vi "Field Transform Joystick.vi"(7 "use field orientation":bool, 9 "Climber Angle":bool, 10 "robot field orientation (deg)":dbl, 11 "Joystick Values":dbl[](array[numeric])) -> (3 "Transformed Joystick Values":dbl[](array[numeric]))   [LabVIEW 2019]
uses:
  <vilib>/Analysis/coordinate.llb/2D Cartesian Coordinate Rotation (Scalar).vi
  <vilib>/addons/control/pid/pid.llb/PID (DBL).vi
  <vilib>/Rock Robotics/Network Tables/NT Write Boolean.vi
  <vilib>/Analysis/NI_AALPro.lvlib
  <vilib>/addons/control/pid/NI_PID_pid.lvlib
panel:
  in  "PID gains":T1={"proportional gain (Kc)"=0.04, "integral time (Ti, min)"=0.0, "derivative time (Td, min)"=0.0} {"derivative time (Td, min)" format="%.3f"; "integral time (Ti, min)" format="%.3f"; "proportional gain (Kc)" format="%.3f"}
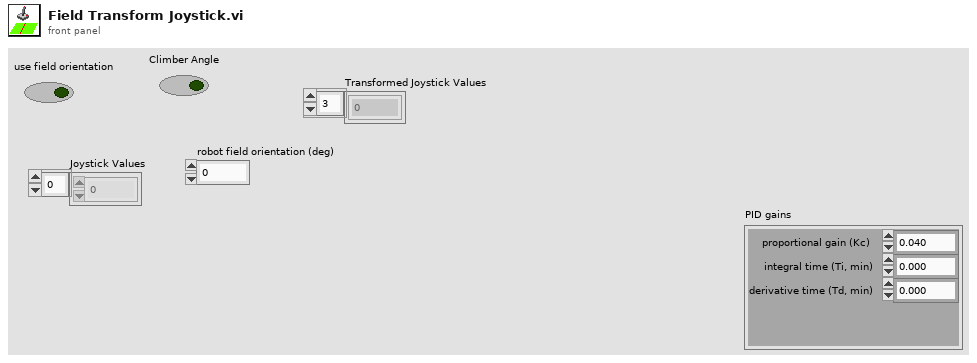
[diagram p1: front panel]
types:
  T1 = cluster{"proportional gain (Kc)":dbl, "integral time (Ti, min)":dbl, "derivative time (Td, min)":dbl}
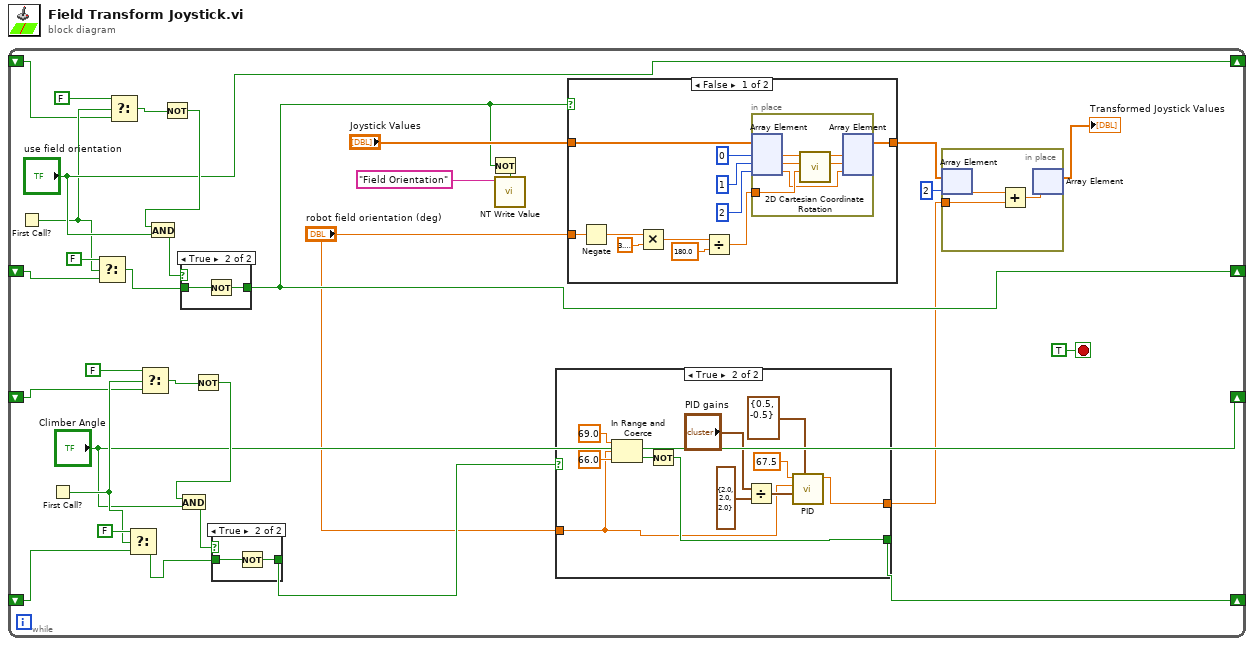
[diagram p0: block diagram]
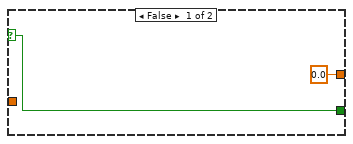
[diagram p2: hidden frame]
diagram:
  n1 = while {
    shift-right: ["use field orientation"] -> _
    shift-left: _ -> [w22]
    shift-right: [w19] -> _
    shift-left: _ -> [w26]
    shift-right: [w6] -> _
    shift-left: _ -> [w9]
    shift-right: ["Climber Angle"] -> _
    shift-left: _ -> [w7]
    stop <- TRUE stop-if-true
    n2 = First Call?() -> (First Call?: T/F=w24:bool)
    n3 = First Call?() -> (First Call?: T/F=w14:bool)
    n4 = Select(t=FALSE, s=w24, f=w26) -> (s? t:f=w20:bool)
    n5 = Select(t=FALSE, s=w24, f=w22) -> (s? t:f=w21:bool)
    n6 = Select(t=FALSE, s=w14, f=w9) -> (s? t:f=w11:bool)
    n7 = Select(t=FALSE, s=w14, f=w7) -> (s? t:f=w12:bool)
    n8 = Not(x=w21) -> (.not. x?=w30:bool)
    n9 = And(x=w30, y="use field orientation") -> (x .and. y?=w28:bool)
    n10 = case shown="True" w28 {
      tunnel: [w52 w54] -> w19
      tunnel: w20 -> [w52 w53]
      frame False {
      }
      frame True {
        n11 = Not(x=w53) -> (.not. x?=w54:bool)
      }
    }
    n12 = Not(x=w12) -> (.not. x?=w17:bool)
    n13 = And(x=w17, y="Climber Angle") -> (x .and. y?=w16:bool)
    n14 = case shown="True" w16 {
      tunnel: [w49 w51] -> w10
      tunnel: w11 -> [w49 w50]
      frame False {
      }
      frame True {
        n15 = Not(x=w50) -> (.not. x?=w51:bool)
      }
    }
    n16 = Not(x=w19) -> (.not. x?=w18:bool)
    n17 = call-poly <vilib>:"NT Write Value.vi"("Boolean"=w18, "Name"="Field Orientation") -> ()  [unwired: 9 in, 1 out]
    n18 = case shown="True" w10 {
      selector: w10 -> [w37 _]
      tunnel: [w37 w40] -> w6
      tunnel: [0.0 ("output") w45] -> w2
      tunnel: "robot field orientation (deg)" -> [_ w38]
      frame False {
      }
      frame True {
        n19 = In Range and Coerce(upper limit=69.0, x=w38, lower limit=66.0) -> (In Range?=w39:bool)  [unwired: 1 out]
        n20 = Not(x=w39) -> (.not. x?=w40:bool)
        n21 = Divide(x="PID gains", y=T1 {"proportional gain (Kc)"=2.0, "integral time (Ti, min)"=2.0, "derivative time (Td, min)"=2.0}) -> (x/y=w46:T1)
        n22 = call-poly <vilib>:"PID.vi"("output range"=cluster{"output high":dbl, "output low":dbl} {"output high"=0.5, "output low"=-0.5}, "PID gains"=w46, "process variable"=w38, "setpoint"=67.5) -> ("output"=w45:dbl)  [unwired: 6 in, 1 out]
      }
    }
    n23 = case shown="False" w19 {
      tunnel: "robot field orientation (deg)" -> [w65 _]
      tunnel: [w55 w72] -> w4
      tunnel: "Joystick Values" -> [w56 w72]
      frame False {
        n24 = Negate(x=w65) -> (-x=w60:dbl)
        n25 = Multiply(x=w60, y=3.141592653589793) -> (x*y=w63:dbl)
        n26 = Divide(x=w63, y=180.0) -> (x/y=w61:dbl)
        n27 = in-place {
          in-place-border: w61 -> [w71]
          n28 = in-place-array #1(w56, 0, 1, 2) -> (w70:dbl, w69:dbl, w66:dbl)
          n29 = call-poly <vilib>:"2D Cartesian Coordinate Rotation.vi"("theta"=w71, "y"=w69, "x"=w70) -> ("y out"=w67:dbl, "x out"=w68:dbl)  [unwired: 6 in, 1 out]
          n30 = in-place-array #1(w68, w67, w66) -> (w55:dbl[])  [unwired: 3 out]
        }
      }
      frame True {
      }
    }
    n31 = in-place {
      in-place-border: w2 -> [w33]
      n32 = in-place-array #2(w4, 2) -> (w35:dbl)
      n33 = Add(x=w35, y=w33) -> (x+y=w34:dbl)
      n34 = in-place-array #2(w34) -> (→"Transformed Joystick Values":dbl[])  [unwired: 1 out]
    }
  }
